vi "Shift Registers.vi"() -> ()   [LabVIEW 2023]
panel:
  out "Previous Number":dbl
  out "Numeric":i32
  in  "stop":bool
  out "number (0 to 1)":dbl
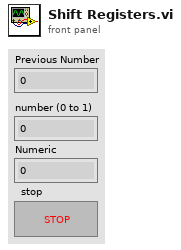
[diagram p1: front panel]
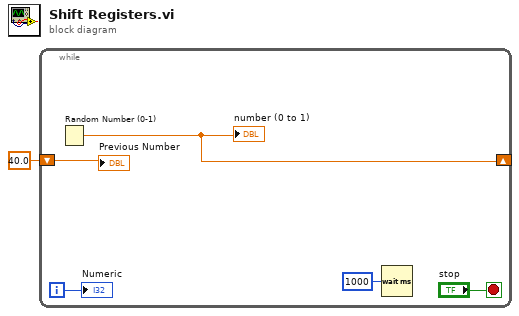
[diagram p0: block diagram]
diagram:
  n1 = while {
    shift-right: [w3] -> _
    shift-left: 40.0 ("number: 0 to 1") -> [w2]
    i -> [w5]
    stop <- "stop" stop-if-true
    n2 = Random Number (0-1)() -> (number: 0 to 1=w3:dbl)
    "number (0 to 1)" <- w3
    n3 = Wait (ms)(milliseconds to wait=u32 1000) -> ()  [unwired: 1 out]
    "Numeric" <- w5
    "Previous Number" <- w2
  }
